vi "TDC_getChannelsEnabled.vi"(8 "Error In":errorcluster) -> (0 "Error Out":errorcluster, 2 "Channel Mask":i32)   [LabVIEW 2011]
uses:
  tdcbase.dll
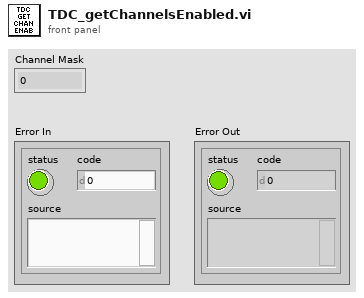
[diagram p1: front panel]
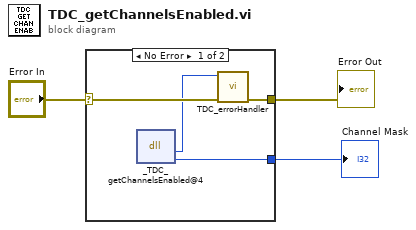
[diagram p0: block diagram]
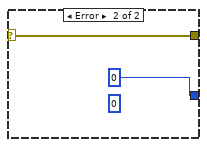
[diagram p2: hidden frame]
diagram:
  n1 = case shown="No Error" "Error In" {
    selector: "Error In" -> [w6 w9]
    tunnel: [w5 w9] -> w2
    tunnel: [w7 0] -> w1
    frame No Error {
      n2 = dll-call lib="X:/tdcbase.dll" fn="_TDC_getChannelsEnabled@4"() -> ("return type"=w4:i32, "chMask"=w7:i32)  [unwired: 4 in, 2 out]
      n3 = call "TDC_errorHandler.vi"("Error In"=w6, "TDC Return Code"=w4) -> ("Error Out"=w5:errorcluster)  [unwired: 9 in]
    }
    frame Error {
      (unwired) 0
    }
  }
  "Error Out" <- w2
  "Channel Mask" <- w1
